vi "map.vi"(1 "Cluster 2":T1) -> (0 "new picture":picture)   [LabVIEW 2014]
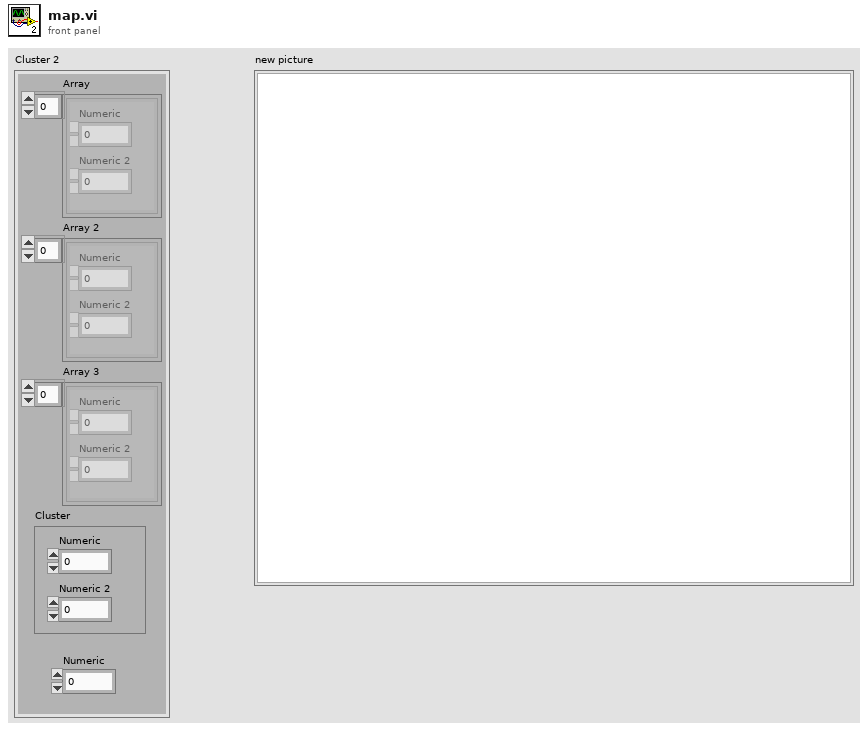
[diagram p1: front panel]
types:
  T1 = cluster{"Array":cluster{"Numeric":dbl, "Numeric 2":dbl}[], "Array 2":cluster{"Numeric":dbl, "Numeric 2":dbl}[], "Array 3":cluster{"Numeric":dbl, "Numeric 2":dbl}[], "Cluster":cluster{"Numeric":dbl, "Numeric 2":dbl}, "Numeric":dbl}
  T2 = cluster{"Width":i16, "Style":enum32{"Solid", "Dash", "Dot", "DashDot", "DashDotDot"}}
  T3 = cluster{"Numeric":dbl, "Numeric 2":dbl, dbl, dbl}
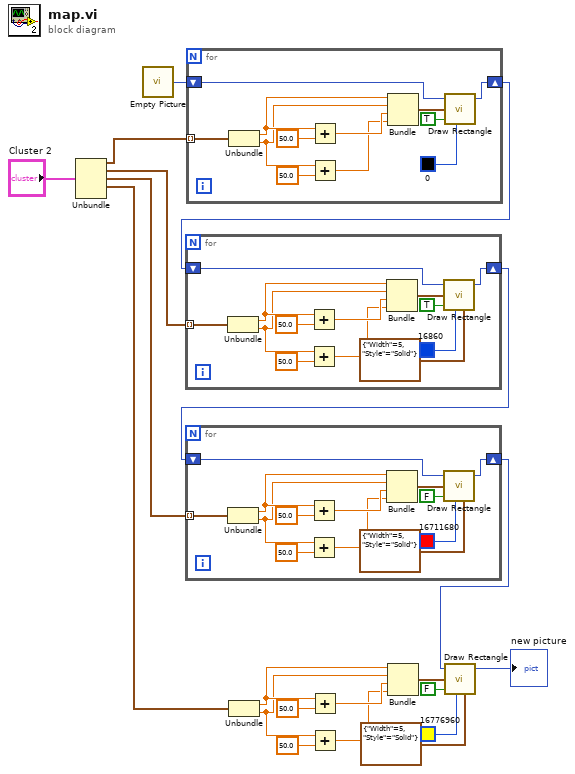
[diagram p0: block diagram]
diagram:
  n1 = Unbundle("Cluster 2") -> ("Array"=w19:cluster{"Numeric":dbl, "Numeric 2":dbl}[], "Array 2"=w17:cluster{"Numeric":dbl, "Numeric 2":dbl}[], "Array 3"=w15:cluster{"Numeric":dbl, "Numeric 2":dbl}[], "Cluster"=w3:cluster{"Numeric":dbl, "Numeric 2":dbl})  [unwired: 1 out]
  n2 = call "Empty Picture"() -> ("empty picture"=w18:picture)
  n3 = for {
    tunnel: w19 -> [w32] mode=indexing
    shift-right: [w21] -> w16
    shift-left: w18 -> [w24]
    n4 = Unbundle(w32) -> ("Numeric"=w29:dbl, "Numeric 2"=w28:dbl)
    n5 = Add(x=w29, y=50.0) -> (x+y=w27:dbl)
    n6 = Add(x=w28, y=50.0) -> (x+y=w26:dbl)
    n7 = Bundle("Numeric"=w29, "Numeric 2"=w28, w27, w26) -> (w25:T3)  [unwired: 1 in]
    n8 = call <vilib>:"Draw Rectangle.vi"("picture"=w24, "rect"=w25, "fill?(F)"=TRUE, "color(black)"=u32 0) -> ("new picture"=w21:picture)  [unwired: 5 in]
  }
  n9 = for {
    tunnel: w17 -> [w45] mode=indexing
    shift-right: [w34] -> w14
    shift-left: w16 -> [w37]
    n10 = Unbundle(w45) -> ("Numeric"=w42:dbl, "Numeric 2"=w41:dbl)
    n11 = Add(x=w42, y=50.0) -> (x+y=w40:dbl)
    n12 = Add(x=w41, y=50.0) -> (x+y=w39:dbl)
    n13 = Bundle("Numeric"=w42, "Numeric 2"=w41, w40, w39) -> (w38:T3)  [unwired: 1 in]
    n14 = call <vilib>:"Draw Rectangle.vi"("picture"=w37, "rect"=w38, "fill?(F)"=TRUE, "color(black)"=u32 16860, "pen"=T2 {"Width"=5, "Style"=enum."Solid"}) -> ("new picture"=w34:picture)  [unwired: 4 in]
  }
  n15 = for {
    tunnel: w15 -> [w58] mode=indexing
    shift-right: [w47] -> w2
    shift-left: w14 -> [w50]
    n16 = Unbundle(w58) -> ("Numeric"=w55:dbl, "Numeric 2"=w54:dbl)
    n17 = Add(x=w55, y=50.0) -> (x+y=w53:dbl)
    n18 = Add(x=w54, y=50.0) -> (x+y=w52:dbl)
    n19 = Bundle("Numeric"=w55, "Numeric 2"=w54, w53, w52) -> (w51:T3)  [unwired: 1 in]
    n20 = call <vilib>:"Draw Rectangle.vi"("picture"=w50, "rect"=w51, "fill?(F)"=FALSE, "color(black)"=u32 16711680, "pen"=T2 {"Width"=5, "Style"=enum."Solid"}) -> ("new picture"=w47:picture)  [unwired: 4 in]
  }
  n21 = Unbundle(w3) -> ("Numeric"=w11:dbl, "Numeric 2"=w10:dbl)
  n22 = Add(x=w11, y=50.0) -> (x+y=w9:dbl)
  n23 = Add(x=w10, y=50.0) -> (x+y=w8:dbl)
  n24 = Bundle("Numeric"=w11, "Numeric 2"=w10, w9, w8) -> (w7:T3)  [unwired: 1 in]
  n25 = call <vilib>:"Draw Rectangle.vi"("picture"=w2, "rect"=w7, "fill?(F)"=FALSE, "color(black)"=u32 16776960, "pen"=T2 {"Width"=5, "Style"=enum."Solid"}) -> ("new picture"=→"new picture":picture)  [unwired: 4 in]
